vi "Untitled 2.vi"() -> ()   [LabVIEW 2018]
panel:
  in  "Boolean 2":bool
  in  "stop":bool
  out "Boolean":bool
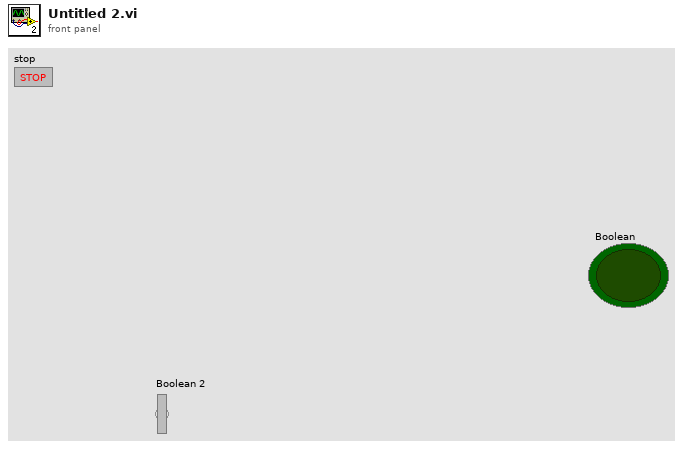
[diagram p1: front panel]
types:
  T1 = cluster{"data[0]":bool, "data[1]":bool, "data[2]":bool, "data[3]":bool, "data[4]":bool, "data[5]":bool, "data[6]":bool, "data[7]":bool, "data[8]":bool}
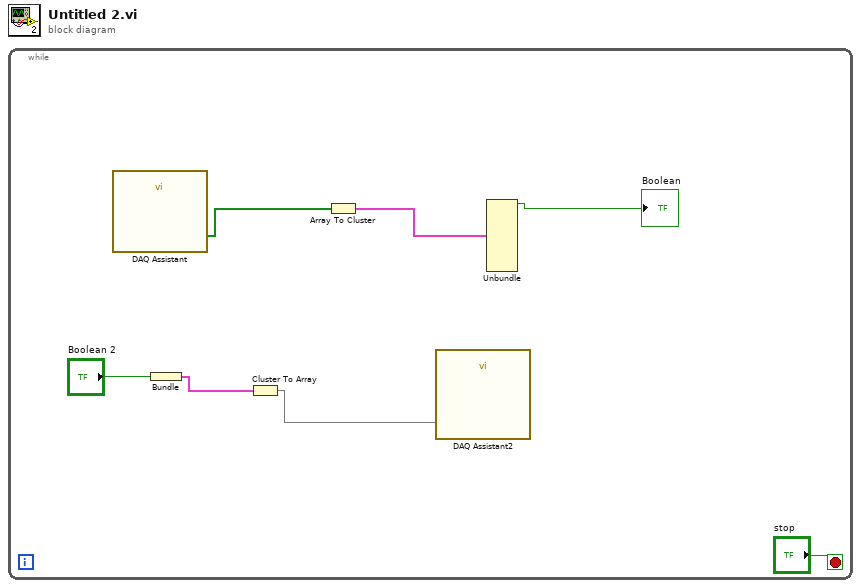
[diagram p0: block diagram]
diagram:
  n1 = while {
    stop <- "stop" stop-if-true
    n2 = call "DAQ Assistant"() -> ("data"=w7:bool[])  [unwired: 17 in, 2 out]
    n3 = Bundle("Boolean 2"="Boolean 2") -> (w3:cluster{"Boolean 2":bool})  [unwired: 1 in]
    n4 = Cluster To Array(cluster=w3) -> (array=w2:bool[])
    n5 = Array To Cluster(array=w7) -> (cluster=w5:T1)
    n6 = call "DAQ Assistant2"("data"=w2) -> ()  [unwired: 17 in, 2 out]
    n7 = Unbundle(w5) -> ("data[0]"=→"Boolean":bool)  [unwired: 8 out]
  }
